vi "Set_Output_State.vi"(7 "Menu Ring":u16(ring) items=["Channel 1", "Channel 2"], 9 "Output State":bool, 11 "VISA resource name":refnum<visa-resource-name>) -> ()   [LabVIEW 2011]
panel:
  out "VISA resource name out":refnum<visa-resource-name>
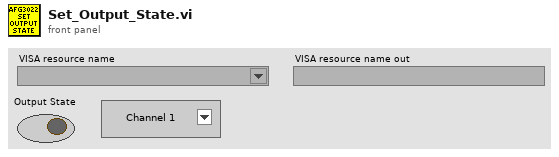
[diagram p1: front panel]
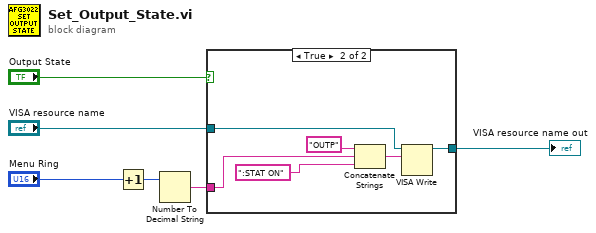
[diagram p0: block diagram]
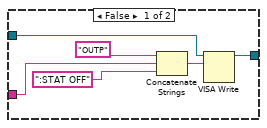
[diagram p2: hidden frame]
diagram:
  n1 = Increment(x="Menu Ring") -> (x+1=w4:u16)
  n2 = Number To Decimal String(number=w4) -> (decimal integer string=w3:string)  [unwired: 1 in]
  n3 = case shown="True" "Output State" {
    tunnel: "VISA resource name" -> [w12 w13]
    tunnel: w3 -> [w10 w15]
    tunnel: [w7 w14] -> w1
    frame False {
      n4 = Concatenate Strings("OUTP" ("write buffer"), w10, ":STAT OFF" ("write buffer")) -> (w8:string)
      n5 = VISA Write(VISA resource name=w12, write buffer=w8) -> (VISA resource name out=w7:refnum<visa-resource-name>)  [unwired: 1 in, 2 out]
    }
    frame True {
      n6 = Concatenate Strings("OUTP" ("write buffer"), w15, ":STAT ON" ("write buffer")) -> (w16:string)
      n7 = VISA Write(VISA resource name=w13, write buffer=w16) -> (VISA resource name out=w14:refnum<visa-resource-name>)  [unwired: 1 in, 2 out]
    }
  }
  "VISA resource name out" <- w1
